vi "LOC subReadWriteVIStringINIKeys(Caption).vi"(4 "Mode":enum16{"Read", "Write"}(ring), 5 "Section":string, 6 "error in (no error)":errorcluster, 8 "ConfigFileRefnum":T1, 9 "ControlRefnum":refnum<vi>) -> (0 "error out":errorcluster, 3 "dup ControlRefnum":refnum<vi>)   [LabVIEW 2020, in "Localization_Tools.lvlib"]
uses:
  Localization_Tools.lvlib
  <vilib>/Utility/config.llb/Config Data RefNum.ctl
  <vilib>/Utility/config.llb/NI_LVConfig.lvlib
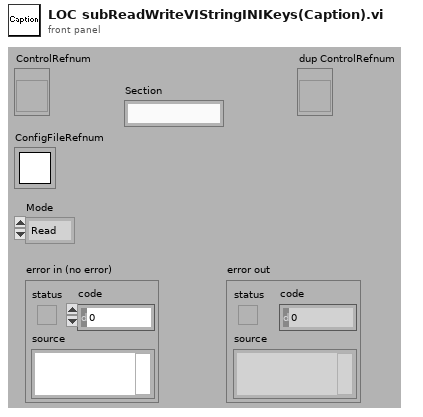
[diagram p1: front panel]
types:
  T1 = typedef "NI_LVConfig.lvlib/Config Data RefNum.ctl" = refnum<k1>
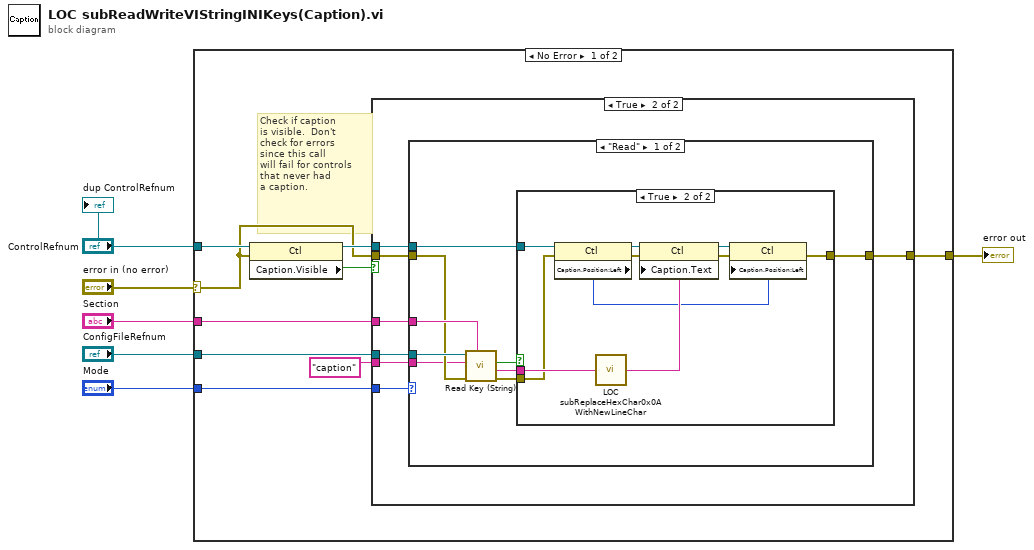
[diagram p0: block diagram]
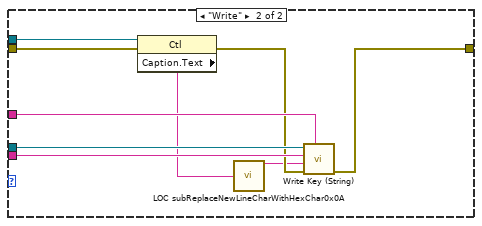
[diagram p4: hidden frame]
diagram:
  n1 = case shown="No Error" "error in (no error)" {
    selector: "error in (no error)" -> [w7 w53]
    tunnel: "Section" -> [w12 _]
    tunnel: "ConfigFileRefnum" -> [w11 _]
    tunnel: "Mode" -> [w10 _]
    tunnel: [w9 w53] -> w3
    tunnel: "ControlRefnum" -> [w8 _]
    frame No Error {
      # "Check if caption\nis visible.  Don't\ncheck for errors\nsince this call\nwill fail for controls\nthat never had\na caption."
      n2 = property class="Ctl"(reference=w8, error in=w7) -> (reference out=w14:refnum<vi>, "Caption.Visible"=w15:bool)  [unwired: 1 out]
      n3 = case shown="True" w15 {
        tunnel: w14 -> [_ w23]
        tunnel: w7 -> [w16 w22]
        tunnel: w10 -> [_ w21]
        tunnel: w11 -> [_ w20]
        tunnel: w12 -> [_ w19]
        tunnel: "caption" ("key") -> [_ w18]
        tunnel: [w16 w17] -> w9
        frame False {
          # "Caption not visible... do nothing"
        }
        frame True {
          n4 = case shown="\"Read\"" w21 {
            tunnel: w23 -> [w30 w52]
            tunnel: w22 -> [w28 w51]
            tunnel: w20 -> [w32 w50]
            tunnel: w19 -> [w31 w48]
            tunnel: w18 -> [w27 w49]
            tunnel: [w26 w46] -> w17
            frame "Read" {
              n5 = call <vilib>:"Read Key (String).vi"("section"=w31, "error in (no error)"=w28, "key"=w27, "refnum"=w32) -> ("error out"=w29:errorcluster, "value"=w25:string, "found?"=w24:bool)  [unwired: 4 in, 1 out]
              n6 = case shown="True" w24 {
                tunnel: w30 -> [_ w41]
                tunnel: w29 -> [w33 w39]
                tunnel: [w33 w35] -> w26
                tunnel: w25 -> [_ w43]
                frame False {
                }
                frame True {
                  n7 = property class="Ctl"(reference=w41, error in=w39) -> (reference out=w40:refnum<vi>, error out=w38:errorcluster, "Caption.Position:Left"=w34:i32)
                  n8 = call "LOC subReplaceHexChar0x0AWithNewLineChar.vi"("InputString"=w43) -> ("OutputString"=w42:string)
                  n9 = property class="Ctl"(reference=w40, error in=w38, "Caption.Text"=w42) -> (reference out=w37:refnum<vi>, error out=w36:errorcluster)
                  n10 = property class="Ctl"(reference=w37, error in=w36, "Caption.Position:Left"=w34) -> (error out=w35:errorcluster)  [unwired: 1 out]
                }
              }
            }
            frame "Write" {
              n11 = property class="Ctl"(reference=w52, error in=w51) -> (error out=w47:errorcluster, "Caption.Text"=w45:string)  [unwired: 1 out]
              n12 = call "LOC subReplaceNewLineCharWithHexChar0x0A.vi"("InputString"=w45) -> ("OutputString"=w44:string)
              n13 = call <vilib>:"Write Key (String).vi"("section"=w48, "error in (no error)"=w47, "value"=w44, "key"=w49, "refnum"=w50) -> ("error out"=w46:errorcluster)  [unwired: 4 in, 2 out]
            }
          }
        }
      }
    }
    frame Error {
    }
  }
  "error out" <- w3
  "dup ControlRefnum" <- "ControlRefnum"
